vi "CreateClass.vi"(7 "PythonConverter_BD in":refnum<class "PyConvBD.lvclass">, 8 "error in":errorcluster, 11 "GObject in":refnum<class "GObject.lvclass">) -> (0 "error out":errorcluster, 3 "GObject out":refnum<class "GObject.lvclass">, 4 "class":string, 5 "PythonConverter_BD out":refnum<class "PyConvBD.lvclass">)   [LabVIEW 2014, in "GObject.lvclass"]
uses:
  GObject.lvclass
  Python/PythonConverter_BD/PyConvBD.lvclass
  Python/Parsing/ClassTypeTD.ctl
  Python/Parsing/Python Functions.lvlib
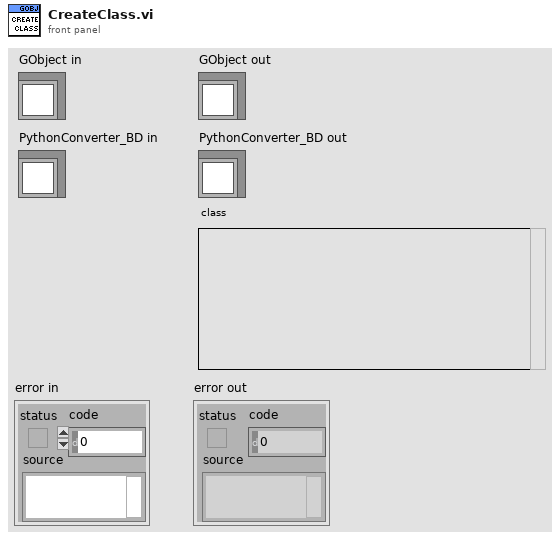
[diagram p1: front panel]
types:
  T1 = typedef "Python Functions.lvlib/ClassTypeTD.ctl" = enum16{"class", "function"}
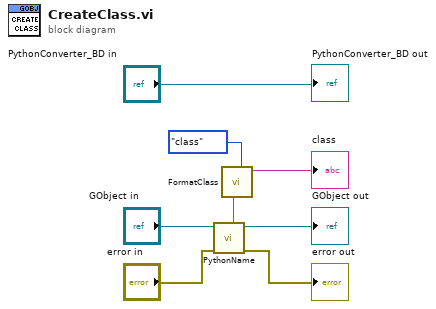
[diagram p0: block diagram]
diagram:
  n1 = call-dynamic "PythonName.vi"("error in"="error in", "GObject in"="GObject in") -> ("error out"=→"error out":errorcluster, "GObject out"=→"GObject out":refnum<class "GObject.lvclass">, "name"=w4:string)  [unwired: 6 in, 1 out]
  n2 = call "FormatClass.vi"("type"=ClassTypeTD."class", "name"=w4) -> ("python"=→"class":string)  [unwired: 9 in]
  "PythonConverter_BD out" <- "PythonConverter_BD in"
